vi "MultiStringToNumberDelimiterSemicolumn.vi"(8 "input string 4":string, 9 "input string 3":string, 10 "input string 2":string, 11 "input string":string) -> (0 "number 4":i32, 1 "number 3":i32, 2 "number 2":i32, 3 "number":i32)   [LabVIEW 2012]
uses:
  <vilib>/regexp/Match Regular Expression.xnode
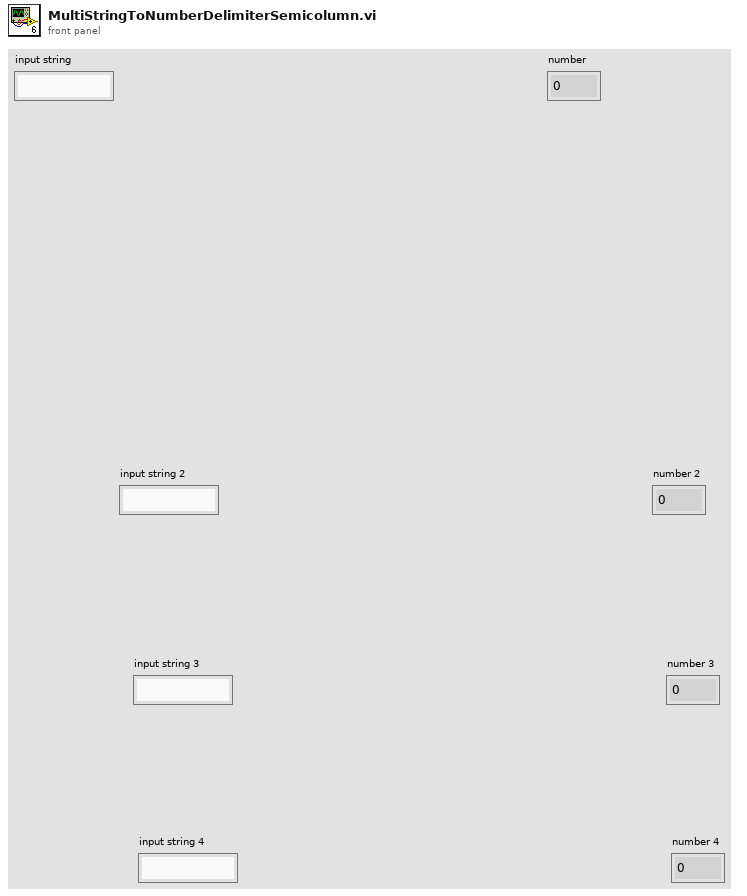
[diagram p1: front panel]
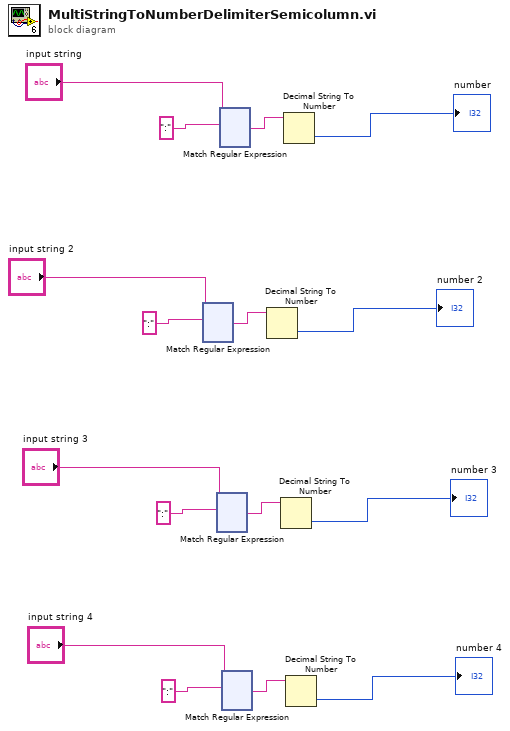
[diagram p0: block diagram]
diagram:
  n1 = xnode "Match Regular Expression"("input string"="input string 2", "regular expression"=":") -> ("after match"=w10:string)  [unwired: 4 in, 4 out]
  n2 = xnode "Match Regular Expression"("input string"="input string 3", "regular expression"=":") -> ("after match"=w6:string)  [unwired: 4 in, 4 out]
  n3 = xnode "Match Regular Expression"("input string"="input string", "regular expression"=":") -> ("after match"=w14:string)  [unwired: 4 in, 4 out]
  n4 = xnode "Match Regular Expression"("input string"="input string 4", "regular expression"=":") -> ("after match"=w2:string)  [unwired: 4 in, 4 out]
  n5 = Decimal String To Number(string=w10) -> (number=→"number 2":i32)  [unwired: 2 in, 1 out]
  n6 = Decimal String To Number(string=w6) -> (number=→"number 3":i32)  [unwired: 2 in, 1 out]
  n7 = Decimal String To Number(string=w14) -> (number=→"number":i32)  [unwired: 2 in, 1 out]
  n8 = Decimal String To Number(string=w2) -> (number=→"number 4":i32)  [unwired: 2 in, 1 out]
